vi "Cache.Result.Read.vi"(7 "Idx":i32, 8 "error in (no error)":errorcluster, 11 "ResultsPath":path=path "D:/svn/LineTraceSystem/SOFTWARE/logs/results") -> (0 "error out":errorcluster, 1 "ProductComponent":T1, 2 "Result":T2)   [LabVIEW 2016]
uses:
  Cache.TestSteps.Fglb.ResultData.ctl
  Database/ProdaNG/Controls/ProdaNG.ProcessResult.ctl
  Database/ProdaNG/Controls/ProdaNG.ProcessStepResult.ctl
  Database/ProdaNG/Controls/ProdaNG.TestStepResult.ctl
  Database/ProdaNG/Controls/ProdaNG.TestValueResult.ctl
  Database/ProdaNG/Controls/ProdaNG.ProductComponent.ctl
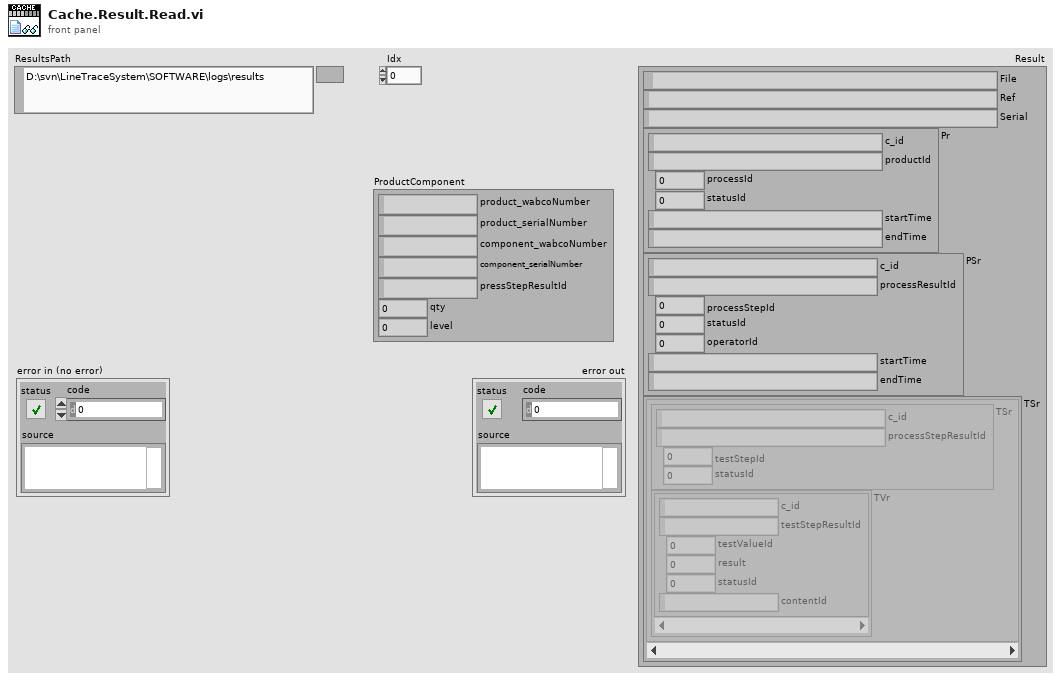
[diagram p1: front panel]
types:
  T1 = typedef "ProdaNG.ProductComponent.ctl" = cluster{"product_wabcoNumber":string, "product_serialNumber":string, "component_wabcoNumber":string, "component_serialNumber":string, "pressStepResultId":string, "qty":i32, "level":i32}
  T2 = typedef "Cache.TestSteps.Fglb.ResultData.ctl" = cluster{"File":path, "Ref":string, "Serial":string, "Pr":T3, "PSr":T4, "TSr":cluster{"TSr":T5, "TVr":T6[]}[]}
  T3 = typedef "ProdaNG.ProcessResult.ctl" = cluster{"c_id":string, "productId":string, "processId":i32, "statusId":i32, "startTime":string, "endTime":string}
  T4 = typedef "ProdaNG.ProcessStepResult.ctl" = cluster{"c_id":string, "processResultId":string, "processStepId":i32, "statusId":i32, "operatorId":i32, "startTime":string, "endTime":string}
  T5 = typedef "ProdaNG.TestStepResult.ctl" = cluster{"c_id":string, "processStepResultId":string, "testStepId":i32, "statusId":i32}
  T6 = typedef "ProdaNG.TestValueResult.ctl" = cluster{"c_id":string, "testStepResultId":string, "testValueId":i32, "result":dbl, "statusId":i32, "contentId":string}
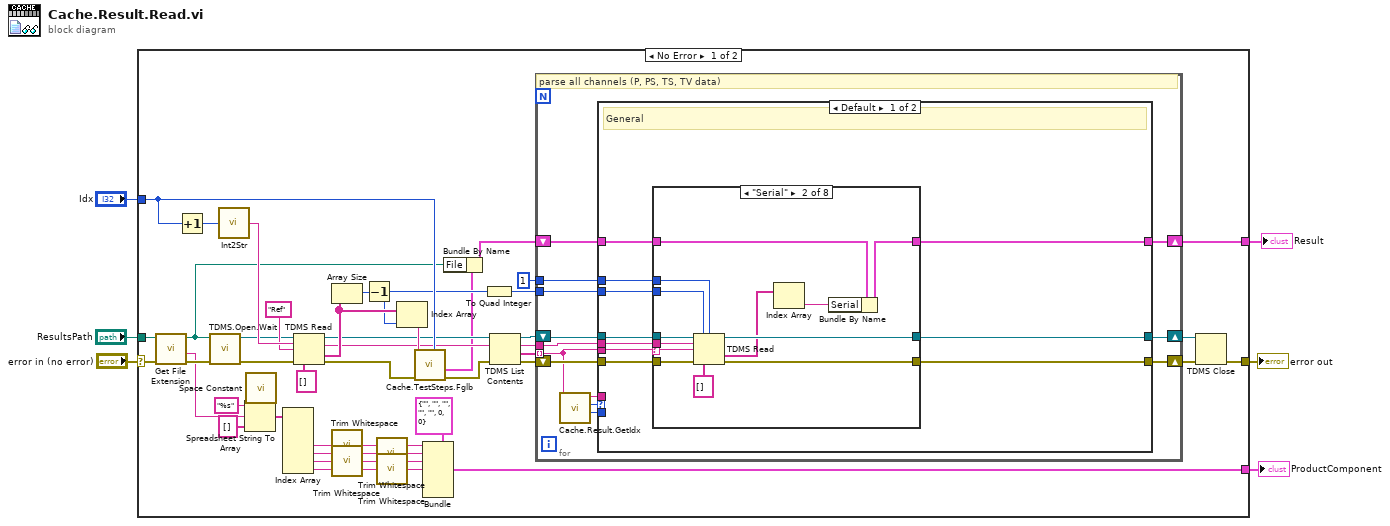
[diagram p0: block diagram]
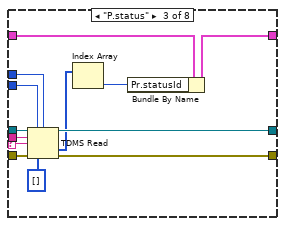
[diagram p3: hidden frame]
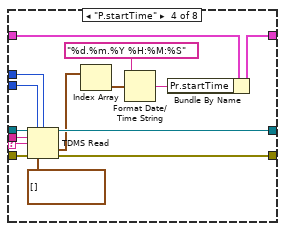
[diagram p4: hidden frame]
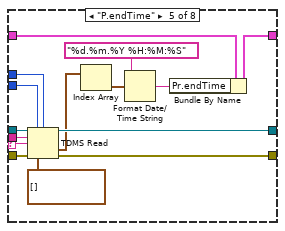
[diagram p5: hidden frame]
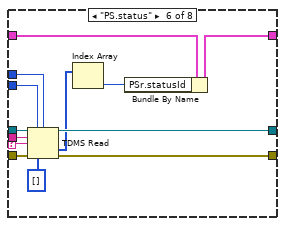
[diagram p6: hidden frame]
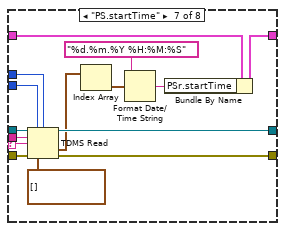
[diagram p7: hidden frame]
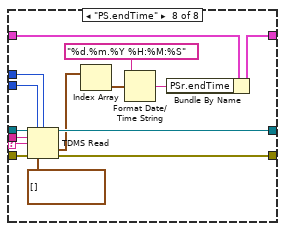
[diagram p8: hidden frame]
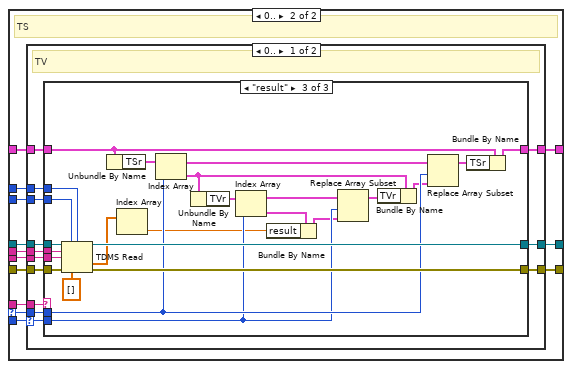
[diagram p9: hidden frame]
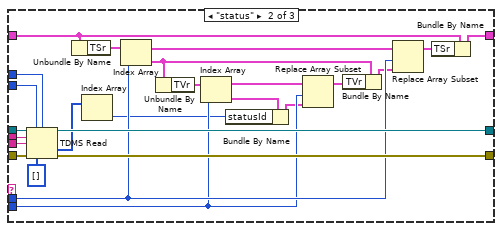
[diagram p11: hidden frame]
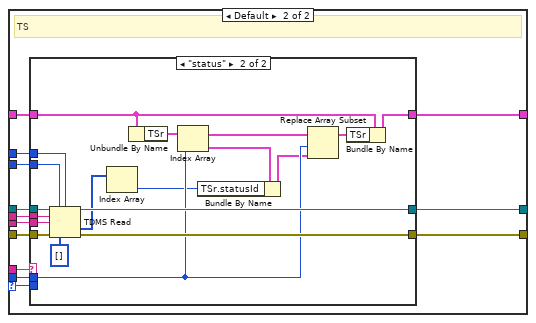
[diagram p12: hidden frame]
diagram:
  n1 = case shown="No Error" "error in (no error)" {
    selector: "error in (no error)" -> [w17 w286]
    tunnel: [w51 w286] -> w6
    tunnel: "ResultsPath" -> [w18 _]
    tunnel: "Idx" -> [w41 _]
    tunnel: [w44 _] -> w2
    tunnel: [w11 _] -> w1
    frame No Error {
      n2 = call <vilib>:"Get File Extension.vi"("error in (no error)"=w17, "file"=w18) -> ("error out"=w16:errorcluster, "filename without extension"=w9:string, "dup file"=w7:path)  [unwired: 5 in, 2 out]
      n3 = Increment(x=w41) -> (x+1=w28:i32)
      n4 = call "TDMS.Open.Wait.vi"("error in (no error)"=w16, "file path"=w7) -> ("error out"=w42:errorcluster, "tdms file out"=w31:refnum<k34>)  [unwired: 8 in]
      n5 = call "Int2Str.vi"("Numeric"=w28) -> ("string"=w40:string)
      n6 = call <vilib>:"Space Constant.vi"() -> ("String"=w26:string)
      n7 = Spreadsheet String To Array(delimiter (Tab)=w26, format string="%s", spreadsheet string=w9, array type (2D Dbl)=string[] []) -> (array=w24:string[])
      n8 = Index Array(array=w24) -> (element #3=w22:string, element #4=w21:string, element #5=w20:string, element #6=w19:string)  [unwired: 6 in, 2 out]
      n9 = TDMS Read(0:w31, 5:w40, 7:"Ref", 11:w42, 12:string[] []) -> (4:w30:refnum<k34>, 6:w32:string, 10:w36:string[], 15:w33:errorcluster)  [unwired: 3 in, 2 out]
      n10 = Array Size(array=w36) -> (size(s)=w37:i32)
      n11 = call <vilib>:"Trim Whitespace.vi"("string"=w22) -> ("trimmed string"=w15:string)  [unwired: 1 in]
      n12 = call <vilib>:"Trim Whitespace.vi"("string"=w20) -> ("trimmed string"=w13:string)  [unwired: 1 in]
      n13 = Decrement(x=w37) -> (x-1=w35:i32)
      n14 = call <vilib>:"Trim Whitespace.vi"("string"=w21) -> ("trimmed string"=w14:string)  [unwired: 1 in]
      n15 = call <vilib>:"Trim Whitespace.vi"("string"=w19) -> ("trimmed string"=w12:string)  [unwired: 1 in]
      n16 = Index Array(array=w36, index=w35) -> (element=w34:string)
      n17 = call "Cache.TestSteps.Fglb.vi"("SystemIdx"=w41, "error in (no error)"=w33, "Variant"=w34) -> ("error out"=w50:errorcluster, "Result out"=w10:T2)  [unwired: 5 in, 2 out]
      n18 = Bundle(cluster=T1 {"product_wabcoNumber"="", "product_serialNumber"="", "component_wabcoNumber"="", "component_serialNumber"="", "pressStepResultId"="", "qty"=0, "level"=0} ("ProductComponent"), "product_wabcoNumber"=w15, "product_serialNumber"=w14, "component_wabcoNumber"=w13, "component_serialNumber"=w12) -> (w11:T1)  [unwired: 3 in]
      n19 = Bundle By Name(cluster=w10, "File"=w7) -> (w8:T2)
      n20 = To Quad Integer(1:w35) -> (0:w29:i64)
      n21 = TDMS List Contents(4:w50, 6:w32, 7:w30) -> (0:w46:errorcluster, 1:w47:string[], 2:w49:string, 3:w48:refnum<k34>)
      n22 = for {
        shift-right: [w61] -> w43
        shift-left: w46 -> [w64]
        shift-right: [w59] -> _
        shift-left: w48 -> [w63]
        tunnel: w47 -> [w54] mode=indexing
        tunnel: w49 -> [w62]
        tunnel: i64 1 ("64bit integer") -> [w60]
        shift-right: [w57] -> w44
        shift-left: w8 -> [w58]
        tunnel: w29 -> [w52]
        # "parse all channels (P, PS, TS, TV data)"
        n23 = call "Cache.Result.GetIdx.vi"("String"=w54) -> ("TV idx"=w55:i32, "TS idx"=w56:i32, "remaining string"=w53:string)  [unwired: 8 in]
        n24 = case shown="Default" w56 {
          selector: w56 -> [_ w180]
          tunnel: w55 -> [_ w179]
          tunnel: w64 -> [w74 w189]
          tunnel: w54 -> [w73 w188]
          tunnel: w63 -> [w71 w187]
          tunnel: w62 -> [w72 w186]
          tunnel: [w70 w185] -> w61
          tunnel: w60 -> [w67 w184]
          tunnel: [w69 w183] -> w59
          tunnel: w58 -> [w68 w182]
          tunnel: [w66 w181] -> w57
          tunnel: w53 -> [_ w178]
          tunnel: w52 -> [w65 w177]
          frame Default {
            # "General"
            n25 = case shown="\"Serial\"" w73 {
              selector: w73 -> [_ w87 w100 w115 w130 w143 w158 w173]
              tunnel: w74 -> [w75 w90 w103 w118 w133 w146 w161 w176]
              tunnel: w71 -> [w76 w89 w102 w117 w132 w145 w160 w175]
              tunnel: w72 -> [_ w88 w101 w116 w131 w144 w159 w174]
              tunnel: [w75 w86 w99 w114 w129 w142 w157 w172] -> w70
              tunnel: w67 -> [_ w85 w98 w113 w128 w141 w156 w171]
              tunnel: [w76 w84 w97 w112 w127 w140 w155 w170] -> w69
              tunnel: w68 -> [w77 w80 w93 w106 w121 w136 w149 w164]
              tunnel: [w77 w79 w92 w105 w120 w135 w148 w163] -> w66
              tunnel: w65 -> [_ w78 w91 w104 w119 w134 w147 w162]
              frame Default {
              }
              frame "Serial" {
                n26 = TDMS Read(0:w89, 1:w78, 2:w85, 5:w88, 7:w87, 11:w90, 12:string[] []) -> (4:w84:refnum<k34>, 10:w82:string[], 15:w86:errorcluster)  [unwired: 1 in, 3 out]
                n27 = Index Array(array=w82) -> (element=w81:string)  [unwired: 1 in]
                n28 = Bundle By Name(cluster=w80, "Serial"=w81) -> (w79:T2)
              }
              frame "P.status" {
                n29 = TDMS Read(0:w102, 1:w91, 2:w98, 5:w101, 7:w100, 11:w103, 12:i32[] []) -> (4:w97:refnum<k34>, 10:w95:i32[], 15:w99:errorcluster)  [unwired: 1 in, 3 out]
                n30 = Index Array(array=w95) -> (element=w94:i32)  [unwired: 1 in]
                n31 = Bundle By Name(cluster=w93, "Pr.statusId"=w94) -> (w92:T2)
              }
              frame "P.startTime" {
                n32 = TDMS Read(0:w117, 1:w104, 2:w113, 5:w116, 7:w115, 11:w118, 12:timestamp[] []) -> (4:w112:refnum<k34>, 10:w108:timestamp[], 15:w114:errorcluster)  [unwired: 1 in, 3 out]
                n33 = Index Array(array=w108) -> (element=w107:timestamp)  [unwired: 1 in]
                n34 = Format Date/Time String(time format string (%c)="%d.%m.%Y %H:%M:%S", seconds (now)=w107) -> (date/time string=w109:string)  [unwired: 1 in]
                n35 = Bundle By Name(cluster=w106, "Pr.startTime"=w109) -> (w105:T2)
              }
              frame "P.endTime" {
                n36 = TDMS Read(0:w132, 1:w119, 2:w128, 5:w131, 7:w130, 11:w133, 12:timestamp[] []) -> (4:w127:refnum<k34>, 10:w123:timestamp[], 15:w129:errorcluster)  [unwired: 1 in, 3 out]
                n37 = Index Array(array=w123) -> (element=w122:timestamp)  [unwired: 1 in]
                n38 = Format Date/Time String(time format string (%c)="%d.%m.%Y %H:%M:%S", seconds (now)=w122) -> (date/time string=w124:string)  [unwired: 1 in]
                n39 = Bundle By Name(cluster=w121, "Pr.endTime"=w124) -> (w120:T2)
              }
              frame "PS.status" {
                n40 = TDMS Read(0:w145, 1:w134, 2:w141, 5:w144, 7:w143, 11:w146, 12:i32[] []) -> (4:w140:refnum<k34>, 10:w138:i32[], 15:w142:errorcluster)  [unwired: 1 in, 3 out]
                n41 = Index Array(array=w138) -> (element=w137:i32)  [unwired: 1 in]
                n42 = Bundle By Name(cluster=w136, "PSr.statusId"=w137) -> (w135:T2)
              }
              frame "PS.startTime" {
                n43 = TDMS Read(0:w160, 1:w147, 2:w156, 5:w159, 7:w158, 11:w161, 12:timestamp[] []) -> (4:w155:refnum<k34>, 10:w151:timestamp[], 15:w157:errorcluster)  [unwired: 1 in, 3 out]
                n44 = Index Array(array=w151) -> (element=w150:timestamp)  [unwired: 1 in]
                n45 = Format Date/Time String(time format string (%c)="%d.%m.%Y %H:%M:%S", seconds (now)=w150) -> (date/time string=w152:string)  [unwired: 1 in]
                n46 = Bundle By Name(cluster=w149, "PSr.startTime"=w152) -> (w148:T2)
              }
              frame "PS.endTime" {
                n47 = TDMS Read(0:w175, 1:w162, 2:w171, 5:w174, 7:w173, 11:w176, 12:timestamp[] []) -> (4:w170:refnum<k34>, 10:w166:timestamp[], 15:w172:errorcluster)  [unwired: 1 in, 3 out]
                n48 = Index Array(array=w166) -> (element=w165:timestamp)  [unwired: 1 in]
                n49 = Format Date/Time String(time format string (%c)="%d.%m.%Y %H:%M:%S", seconds (now)=w165) -> (date/time string=w167:string)  [unwired: 1 in]
                n50 = Bundle By Name(cluster=w164, "PSr.endTime"=w167) -> (w163:T2)
              }
            }
          }
          frame 0.. {
            # "TS"
            n51 = case shown="0.." w179 {
              selector: w179 -> [w191 w253]
              tunnel: w189 -> [w200 w262]
              tunnel: w188 -> [w197 w259]
              tunnel: w187 -> [w199 w261]
              tunnel: w186 -> [w198 w260]
              tunnel: [w193 w255] -> w185
              tunnel: w177 -> [w196 w258]
              tunnel: w184 -> [w195 w257]
              tunnel: [w194 w256] -> w183
              tunnel: w182 -> [w201 w263]
              tunnel: [w202 w264] -> w181
              tunnel: w180 -> [w192 w254]
              tunnel: w178 -> [w190 w252]
              frame 0.. {
                # "TV"
                n52 = case shown="\"result\"" w190 {
                  tunnel: [w205 w209 w232] -> w202
                  tunnel: w201 -> [w205 w208 w231]
                  tunnel: w200 -> [w203 w228 w251]
                  tunnel: w199 -> [w204 w227 w250]
                  tunnel: w198 -> [_ w226 w249]
                  tunnel: w197 -> [_ w225 w248]
                  tunnel: w196 -> [_ w224 w247]
                  tunnel: w195 -> [_ w223 w246]
                  tunnel: [w204 w221 w244] -> w194
                  tunnel: [w203 w220 w243] -> w193
                  tunnel: w192 -> [_ w219 w242]
                  tunnel: w191 -> [_ w218 w241]
                  frame Default {
                  }
                  frame "status" {
                    n53 = TDMS Read(0:w227, 1:w224, 2:w223, 5:w226, 7:w225, 11:w228, 12:i32[] []) -> (4:w221:refnum<k34>, 10:w207:i32[], 15:w220:errorcluster)  [unwired: 1 in, 3 out]
                    n54 = Unbundle By Name(w208) -> ("TSr"=w212:cluster{"TSr":T5, "TVr":T6[]}[])
                    n55 = Index Array(array=w207) -> (element=w206:i32)  [unwired: 1 in]
                    n56 = Index Array(array=w212, index=w219) -> (element=w213:cluster{"TSr":T5, "TVr":T6[]})
                    n57 = Unbundle By Name(w213) -> ("TVr"=w216:T6[])
                    n58 = Index Array(array=w216, index=w218) -> (element=w217:T6)
                    n59 = Bundle By Name(cluster=w217, "statusId"=w206) -> (w215:T6)
                    n60 = Replace Array Subset(array=w216, new element=w215, index=w218) -> (w214:T6[])
                    n61 = Bundle By Name(cluster=w213, "TVr"=w214) -> (w210:cluster{"TSr":T5, "TVr":T6[]})
                    n62 = Replace Array Subset(array=w212, new element=w210, index=w219) -> (w211:cluster{"TSr":T5, "TVr":T6[]}[])
                    n63 = Bundle By Name(cluster=w208, "TSr"=w211) -> (w209:T2)
                  }
                  frame "result" {
                    n64 = TDMS Read(0:w250, 1:w247, 2:w246, 5:w249, 7:w248, 11:w251, 12:dbl[] []) -> (4:w244:refnum<k34>, 10:w230:dbl[], 15:w243:errorcluster)  [unwired: 1 in, 3 out]
                    n65 = Unbundle By Name(w231) -> ("TSr"=w235:cluster{"TSr":T5, "TVr":T6[]}[])
                    n66 = Index Array(array=w230) -> (element=w229:dbl)  [unwired: 1 in]
                    n67 = Index Array(array=w235, index=w242) -> (element=w236:cluster{"TSr":T5, "TVr":T6[]})
                    n68 = Unbundle By Name(w236) -> ("TVr"=w239:T6[])
                    n69 = Index Array(array=w239, index=w241) -> (element=w240:T6)
                    n70 = Bundle By Name(cluster=w240, "result"=w229) -> (w238:T6)
                    n71 = Replace Array Subset(array=w239, new element=w238, index=w241) -> (w237:T6[])
                    n72 = Bundle By Name(cluster=w236, "TVr"=w237) -> (w233:cluster{"TSr":T5, "TVr":T6[]})
                    n73 = Replace Array Subset(array=w235, new element=w233, index=w242) -> (w234:cluster{"TSr":T5, "TVr":T6[]}[])
                    n74 = Bundle By Name(cluster=w231, "TSr"=w234) -> (w232:T2)
                  }
                }
              }
              frame Default {
                # "TS"
                n75 = case shown="\"status\"" w252 {
                  tunnel: [w267 w270] -> w264
                  tunnel: w263 -> [w267 w271]
                  tunnel: w262 -> [w265 w285]
                  tunnel: w261 -> [w266 w284]
                  tunnel: w260 -> [_ w283]
                  tunnel: w259 -> [_ w282]
                  tunnel: w258 -> [_ w281]
                  tunnel: w257 -> [_ w280]
                  tunnel: [w266 w278] -> w256
                  tunnel: [w265 w277] -> w255
                  tunnel: w254 -> [_ w276]
                  tunnel: w253 -> [_ _]
                  frame Default {
                  }
                  frame "status" {
                    n76 = TDMS Read(0:w284, 1:w281, 2:w280, 5:w283, 7:w282, 11:w285, 12:i32[] []) -> (4:w278:refnum<k34>, 10:w269:i32[], 15:w277:errorcluster)  [unwired: 1 in, 3 out]
                    n77 = Index Array(array=w269) -> (element=w268:i32)  [unwired: 1 in]
                    n78 = Unbundle By Name(w271) -> ("TSr"=w274:cluster{"TSr":T5, "TVr":T6[]}[])
                    n79 = Index Array(array=w274, index=w276) -> (element=w275:cluster{"TSr":T5, "TVr":T6[]})
                    n80 = Bundle By Name(cluster=w275, "TSr.statusId"=w268) -> (w272:cluster{"TSr":T5, "TVr":T6[]})
                    n81 = Replace Array Subset(array=w274, new element=w272, index=w276) -> (w273:cluster{"TSr":T5, "TVr":T6[]}[])
                    n82 = Bundle By Name(cluster=w271, "TSr"=w273) -> (w270:T2)
                  }
                }
              }
            }
          }
        }
      }
      n83 = TDMS Close(8:w43, 11:w30) -> (0:w51:errorcluster)  [unwired: 1 out]
    }
    frame Error {
    }
  }
  "error out" <- w6
  "Result" <- w2
  "ProductComponent" <- w1
